vi "Single Point Wave generation.vi"(11 "Data To Write":i16) -> (3 "error out":errorcluster)   [LabVIEW 2014]
doc: "This VI perform a single write on the DIO from 11 to 23.\nInput is a 12-bit FXP with integer part of 5-bit"
uses:
  <vilib>/rvi/eio/common/nirviEmuTemplateMethod_errors.vi
  <vilib>/eio/EIOMethodNode/EIOMethodNode.xnode
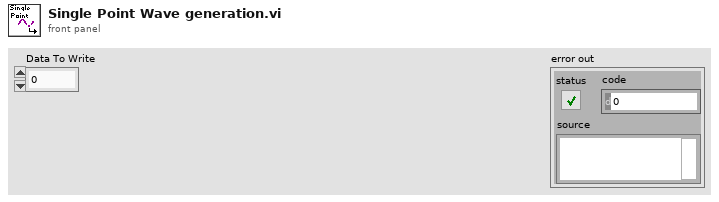
[diagram p1: front panel]
types:
  T1 = cluster{"Boolean array[0]":bool, "Boolean array[1]":bool, "Boolean array[2]":bool, "Boolean array[3]":bool, "Boolean array[4]":bool, "Boolean array[5]":bool, "Boolean array[6]":bool, "Boolean array[7]":bool, "Boolean array[8]":bool, "Boolean array[9]":bool, "Boolean array[10]":bool, "Boolean array[11]":bool}
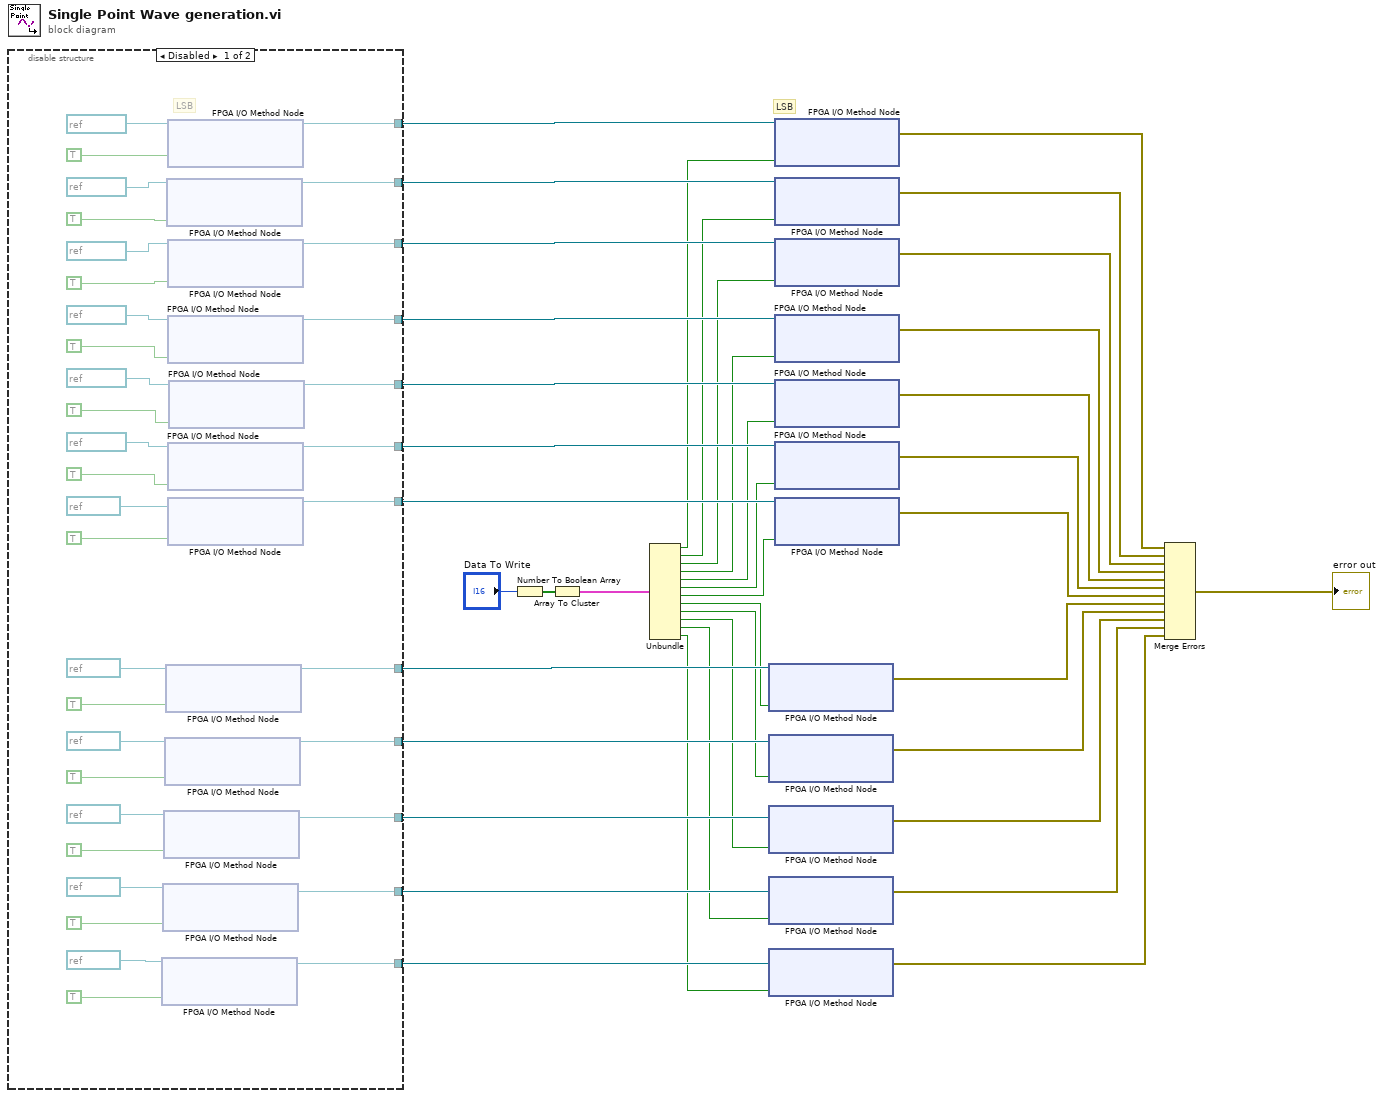
[diagram p0: block diagram]
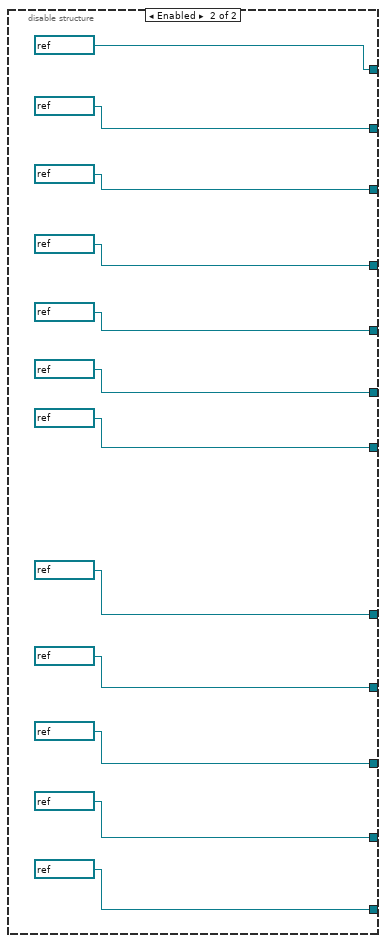
[diagram p2: hidden frame]
diagram:
  # "LSB"
  n1 = disable-structure shown="Disabled" {
    disable-tunnel: [w76 refnum<k21> "DIO12" ("FPGA I/O In")] -> w40
    disable-tunnel: [w74 refnum<k21> "DIO13" ("FPGA I/O In")] -> w39
    disable-tunnel: [w71 refnum<k21> "DIO14" ("FPGA I/O In")] -> w38
    disable-tunnel: [w68 refnum<k21> "DIO15" ("FPGA I/O In")] -> w37
    disable-tunnel: [w65 refnum<k21> "DIO16" ("FPGA I/O In")] -> w36
    disable-tunnel: [w62 refnum<k21> "DIO17" ("FPGA I/O In")] -> w35
    disable-tunnel: [w59 refnum<k21> "DIO18" ("FPGA I/O In")] -> w34
    disable-tunnel: [w56 refnum<k21> "DIO19" ("FPGA I/O In")] -> w33
    disable-tunnel: [w53 refnum<k21> "DIO20" ("FPGA I/O In")] -> w32
    disable-tunnel: [w50 refnum<k21> "DIO21" ("FPGA I/O In")] -> w31
    disable-tunnel: [w47 refnum<k21> "DIO22" ("FPGA I/O In")] -> w30
    disable-tunnel: [w44 refnum<k21> "DIO23" ("FPGA I/O In")] -> w29
    frame Disabled {
      # "LSB"
      n2 = xnode "FPGA I/O Method Node"("FPGA I/O In"=refnum<k21> "DIO4", "Enable"=TRUE) -> ("FPGA I/O Out"=w44:refnum<k21>)
      n3 = xnode "FPGA I/O Method Node"("FPGA I/O In"=refnum<k21> "DIO5", "Enable"=TRUE) -> ("FPGA I/O Out"=w47:refnum<k21>)
      n4 = xnode "FPGA I/O Method Node"("FPGA I/O In"=refnum<k21> "DIO6", "Enable"=TRUE) -> ("FPGA I/O Out"=w50:refnum<k21>)
      n5 = xnode "FPGA I/O Method Node"("FPGA I/O In"=refnum<k21> "DIO7", "Enable"=TRUE) -> ("FPGA I/O Out"=w53:refnum<k21>)
      n6 = xnode "FPGA I/O Method Node"("FPGA I/O In"=refnum<k21> "DIO8", "Enable"=TRUE) -> ("FPGA I/O Out"=w56:refnum<k21>)
      n7 = xnode "FPGA I/O Method Node"("FPGA I/O In"=refnum<k21> "DIO14", "Enable"=TRUE) -> ("FPGA I/O Out"=w74:refnum<k21>)
      n8 = xnode "FPGA I/O Method Node"("FPGA I/O In"=refnum<k21> "DIO15", "Enable"=TRUE) -> ("FPGA I/O Out"=w76:refnum<k21>)
      n9 = xnode "FPGA I/O Method Node"("FPGA I/O In"=refnum<k21> "DIO13", "Enable"=TRUE) -> ("FPGA I/O Out"=w71:refnum<k21>)
      n10 = xnode "FPGA I/O Method Node"("FPGA I/O In"=refnum<k21> "DIO12", "Enable"=TRUE) -> ("FPGA I/O Out"=w68:refnum<k21>)
      n11 = xnode "FPGA I/O Method Node"("FPGA I/O In"=refnum<k21> "DIO10", "Enable"=TRUE) -> ("FPGA I/O Out"=w62:refnum<k21>)
      n12 = xnode "FPGA I/O Method Node"("FPGA I/O In"=refnum<k21> "DIO9", "Enable"=TRUE) -> ("FPGA I/O Out"=w59:refnum<k21>)
      n13 = xnode "FPGA I/O Method Node"("FPGA I/O In"=refnum<k21> "DIO11", "Enable"=TRUE) -> ("FPGA I/O Out"=w65:refnum<k21>)
    }
    frame Enabled {
    }
  }
  n14 = Number To Boolean Array(number="Data To Write") -> (Boolean array=w28:bool[])
  n15 = Array To Cluster(array=w28) -> (cluster=w27:T1)
  n16 = Unbundle(w27) -> ("Boolean array[0]"=w26:bool, "Boolean array[1]"=w25:bool, "Boolean array[2]"=w24:bool, "Boolean array[3]"=w23:bool, "Boolean array[4]"=w22:bool, "Boolean array[5]"=w21:bool, "Boolean array[6]"=w20:bool, "Boolean array[7]"=w19:bool, "Boolean array[8]"=w18:bool, "Boolean array[9]"=w17:bool, "Boolean array[10]"=w16:bool, "Boolean array[11]"=w15:bool)
  n17 = xnode "FPGA I/O Method Node"("FPGA I/O In"=w33, "Data"=w19) -> ("error out"=w6:errorcluster)  [unwired: 1 in, 1 out]
  n18 = xnode "FPGA I/O Method Node"("FPGA I/O In"=w32, "Data"=w18) -> ("error out"=w5:errorcluster)  [unwired: 1 in, 1 out]
  n19 = xnode "FPGA I/O Method Node"("FPGA I/O In"=w31, "Data"=w17) -> ("error out"=w4:errorcluster)  [unwired: 1 in, 1 out]
  n20 = xnode "FPGA I/O Method Node"("FPGA I/O In"=w30, "Data"=w16) -> ("error out"=w3:errorcluster)  [unwired: 1 in, 1 out]
  n21 = xnode "FPGA I/O Method Node"("FPGA I/O In"=w29, "Data"=w15) -> ("error out"=w2:errorcluster)  [unwired: 1 in, 1 out]
  n22 = xnode "FPGA I/O Method Node"("FPGA I/O In"=w40, "Data"=w26) -> ("error out"=w13:errorcluster)  [unwired: 1 in, 1 out]
  n23 = xnode "FPGA I/O Method Node"("FPGA I/O In"=w39, "Data"=w25) -> ("error out"=w12:errorcluster)  [unwired: 1 in, 1 out]
  n24 = xnode "FPGA I/O Method Node"("FPGA I/O In"=w38, "Data"=w24) -> ("error out"=w11:errorcluster)  [unwired: 1 in, 1 out]
  n25 = xnode "FPGA I/O Method Node"("FPGA I/O In"=w37, "Data"=w23) -> ("error out"=w10:errorcluster)  [unwired: 1 in, 1 out]
  n26 = xnode "FPGA I/O Method Node"("FPGA I/O In"=w36, "Data"=w22) -> ("error out"=w9:errorcluster)  [unwired: 1 in, 1 out]
  n27 = xnode "FPGA I/O Method Node"("FPGA I/O In"=w35, "Data"=w21) -> ("error out"=w8:errorcluster)  [unwired: 1 in, 1 out]
  n28 = xnode "FPGA I/O Method Node"("FPGA I/O In"=w34, "Data"=w20) -> ("error out"=w7:errorcluster)  [unwired: 1 in, 1 out]
  n29 = Merge Errors(w13, w12, w11, w10, w9, w8, w7, w6, w5, w4, w3, w2) -> (→"error out":errorcluster)
